vi "Get Component Settings By ID.vi"(8 "error in (no error)":errorcluster, 10 "settings id":T1={"plugin"=-1, "thread"=-1, "group"=-1, "transfer"=-1, "channel"=-1}, 11 "Thread Configuration in":refnum<class "Thread Configuration.lvclass">) -> (0 "error out":errorcluster, 2 "component settings":T2[](array[typedef]), 3 "Thread Configuration out":refnum<class "Thread Configuration.lvclass">)   [LabVIEW 2017, in "DSF Core.lvlib" / "Thread Configuration.lvclass"]
uses:
  Thread Configuration.lvclass
  C:/Git/DSF/Core/Classes/Configuration/Runtime/Runtime Configuration.lvclass
  Typedefs/DSF Settings Info.ctl
  Typedefs/DSF Version Info.ctl
  Typedefs/DSF Configuration ID.ctl
  Thread Configuration.lvclass/Thread Configuration.ctl
  Group/Group Configuration.lvclass
  Runtime/Runtime Configuration.lvclass
  DSF Core.lvlib
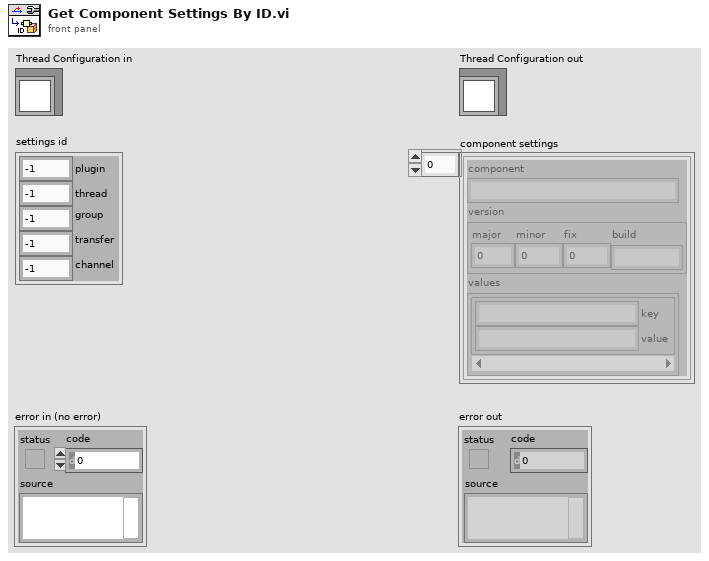
[diagram p1: front panel]
types:
  T1 = typedef "DSF Core.lvlib/DSF Configuration ID.ctl" = cluster{"plugin":i32, "thread":i32, "group":i32, "transfer":i32, "channel":i32}
  T2 = typedef "DSF Core.lvlib/DSF Settings Info.ctl" = cluster{"component":string, "version":T3, "values":cluster{"key":string, "value":string}[]}
  T3 = typedef "DSF Core.lvlib/DSF Version Info.ctl" = cluster{"major":u32, "minor":u32, "fix":u32, "build":string}
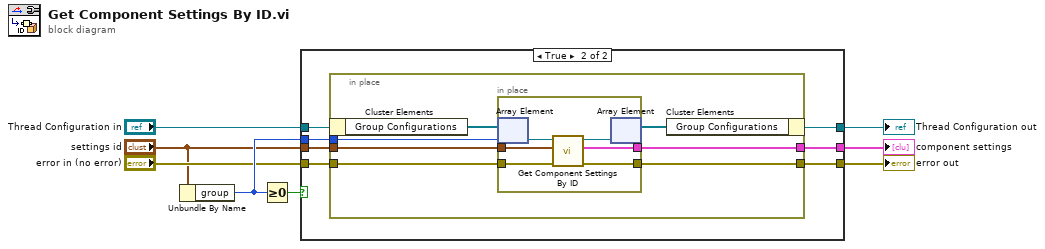
[diagram p0: block diagram]
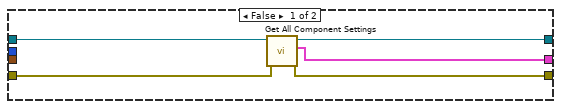
[diagram p2: hidden frame]
diagram:
  n1 = Unbundle By Name("settings id") -> ("group"=w7:i32)
  n2 = Greater Or Equal To 0?(x=w7) -> (x >= 0?=w8:bool)
  n3 = case shown="True" w8 {
    tunnel: [w11 w14] -> w1
    tunnel: w7 -> [_ w16]
    tunnel: "error in (no error)" -> [w12 w20]
    tunnel: [w10 w19] -> w5
    tunnel: [w9 w18] -> w3
    tunnel: "settings id" -> [_ w17]
    tunnel: "Thread Configuration in" -> [w13 w15]
    frame False {
      n4 = call "Get All Component Settings.vi"("error in (no error)"=w12, "Runtime Configuration in"=w13) -> ("error out"=w10:errorcluster, "component settings"=w9:T2[], "Runtime Configuration out"=w11:refnum<class "Thread Configuration.lvclass">)  [unwired: 7 in]
    }
    frame True {
      n5 = in-place {
        in-place-border: w20 -> [w27]
        in-place-border: [w26] -> w19
        in-place-border: [w25] -> w18
        in-place-border: w17 -> [w24]
        in-place-border: w16 -> [w23]
        n6 = in-place-cluster #1(w15) -> ("Group Configurations"=w22:refnum<class "Group Configuration.lvclass">[])
        n7 = in-place {
          in-place-border: w27 -> [w33]
          in-place-border: [w32] -> w26
          in-place-border: [w31] -> w25
          in-place-border: w24 -> [w30]
          n8 = in-place-array #2(w22, w23) -> (w29:refnum<class "Group Configuration.lvclass">)
          n9 = call-dynamic "Get Component Settings By ID.vi"("error in (no error)"=w33, "settings id"=w30, "Group Configuration in"=w29) -> ("error out"=w32:errorcluster, "component settings"=w31:T2[], "Group Configuration out"=w28:refnum<class "Group Configuration.lvclass">)  [unwired: 6 in]
          n10 = in-place-array #2(w28) -> (w21:refnum<class "Group Configuration.lvclass">[])  [unwired: 1 out]
        }
        n11 = in-place-cluster #1("Group Configurations"=w21) -> (w14:refnum<class "Thread Configuration.lvclass">)
      }
    }
  }
  "error out" <- w5
  "Thread Configuration out" <- w1
  "component settings" <- w3
